vi "BRig_Host_dataRunState_dataPlot_init.vi"() -> (2 "output_dataPlot":u16[][](array[numeric]))   [LabVIEW 2014]
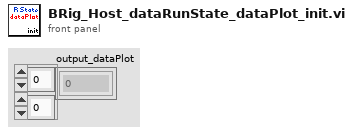
[diagram p1: front panel]
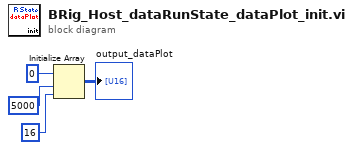
[diagram p0: block diagram]
diagram:
  n1 = Initialize Array(u16 0 ("element"), 5000 ("dimension size"), 16 ("dimension size")) -> (→"output_dataPlot":u16[][])
